vi "adaptTimeStamp.vi"(1 "timestamp in":string) -> (0 "timestamp out":string)   [LabVIEW 2010]
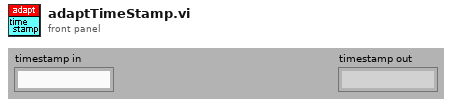
[diagram p1: front panel]
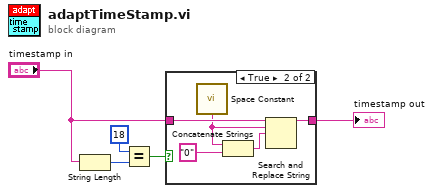
[diagram p0: block diagram]
diagram:
  n1 = String Length(string="timestamp in") -> (length=w4:i32)
  n2 = Equal?(x=18, y=w4) -> (x = y?=w3:bool)
  n3 = case shown="True" w3 {
    tunnel: "timestamp in" -> [w6 w11]
    tunnel: [w6 w10] -> w1
    frame False {
    }
    frame True {
      n4 = call <vilib>:"Space Constant.vi"() -> ("String"=w9:string)
      n5 = Concatenate Strings(w9, "0" ("replace string (\"\")")) -> (w7:string)
      n6 = Search and Replace String(input string=w11, search string=w9, replace string=w7) -> (result string=w10:string)  [unwired: 1 in, 7 out]
    }
  }
  "timestamp out" <- w1
